vi "circle-tsk5.vi"() -> ()   [LabVIEW 2020]
panel:
  in  "r":dbl
  out "XY Graph":cluster{dbl[], dbl[]}[](graph)
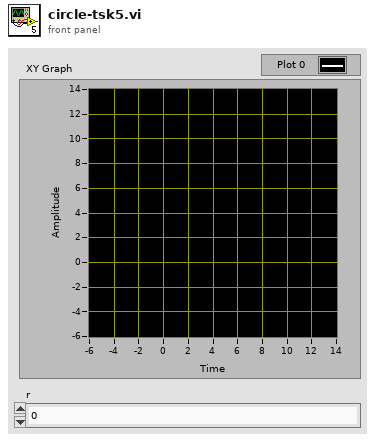
[diagram p1: front panel]
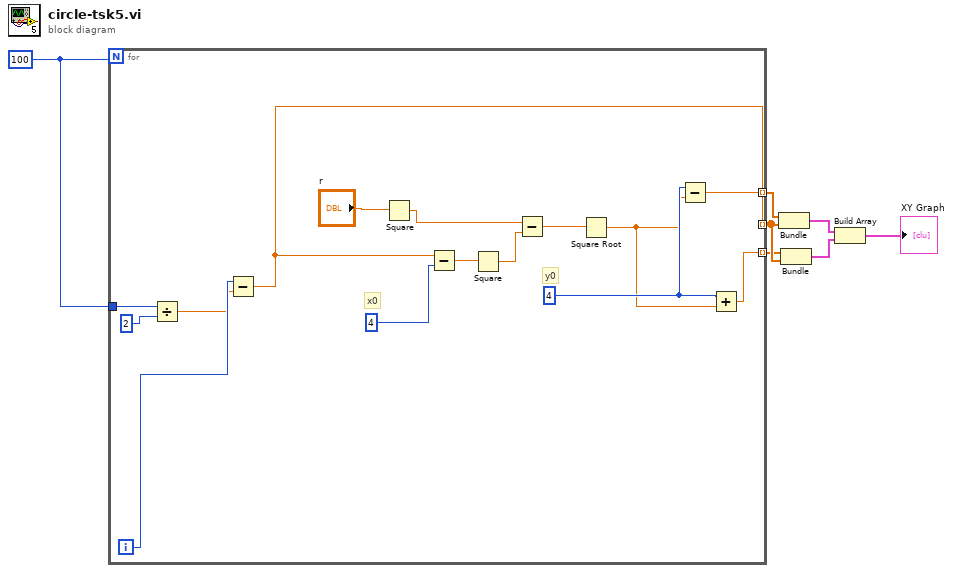
[diagram p0: block diagram]
diagram:
  w7 = 100
  n1 = for {
    N: w7 -> [_]
    tunnel: w7 -> [w21]
    tunnel: [w17] -> w3 mode=indexing
    tunnel: [w9] -> w2 mode=indexing
    tunnel: [w8] -> w1 mode=indexing
    i -> [w20]
    w11 = 4
    # "y0"
    # "x0"
    n2 = Divide(x=w21, y=2) -> (x/y=w19:dbl)
    n3 = Subtract(x=w20, y=w19) -> (x-y=w17:dbl)
    n4 = Square(x="r") -> (x^2=w14:dbl)
    n5 = Subtract(x=w17, y=4) -> (x-y=w15:dbl)
    n6 = Square(x=w15) -> (x^2=w13:dbl)
    n7 = Subtract(x=w14, y=w13) -> (x-y=w12:dbl)
    n8 = Square Root(x=w12) -> (sqrt(x)=w10:dbl)
    n9 = Subtract(x=w11, y=w10) -> (x-y=w9:dbl)
    n10 = Add(x=w11, y=w10) -> (x+y=w8:dbl)
  }
  n11 = Bundle(w2, w3) -> (w6:cluster{dbl[], dbl[]})  [unwired: 1 in]
  n12 = Bundle(w1, w3) -> (w5:cluster{dbl[], dbl[]})  [unwired: 1 in]
  n13 = Build Array(w6, w5) -> (→"XY Graph":cluster{dbl[], dbl[]}[])
